vi "Initialize.vi"(4 "Allow Handler Configuration [F]":bool, 5 "HTTP Client In":refnum<class "HttpClient_NET.lvclass">, 7 "AllowedProtocols":i32[](array[ring]) items=["SystemDefault"=0, "Ssl3"=48, "Tls"=192, "Tls11"=768, "Tls12"=3072, "Tls13"=12288], 8 "error in (no error)":errorcluster) -> (0 "error out":errorcluster, 3 "HTTP Client Out":refnum<class "HttpClient_NET.lvclass">)   [LabVIEW 2018, in "HttpClient_NET.lvlib" / "HttpClient_NET.lvclass"]
uses:
  HttpClient_NET.lvclass
  System.Net.Http
  HttpClient_NET.lvclass/HttpClient_NET.ctl
  Accessors/Write NET_HttpClientHandler.vi
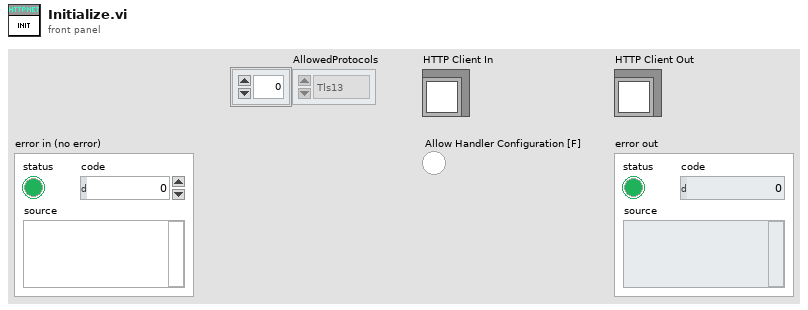
[diagram p1: front panel]
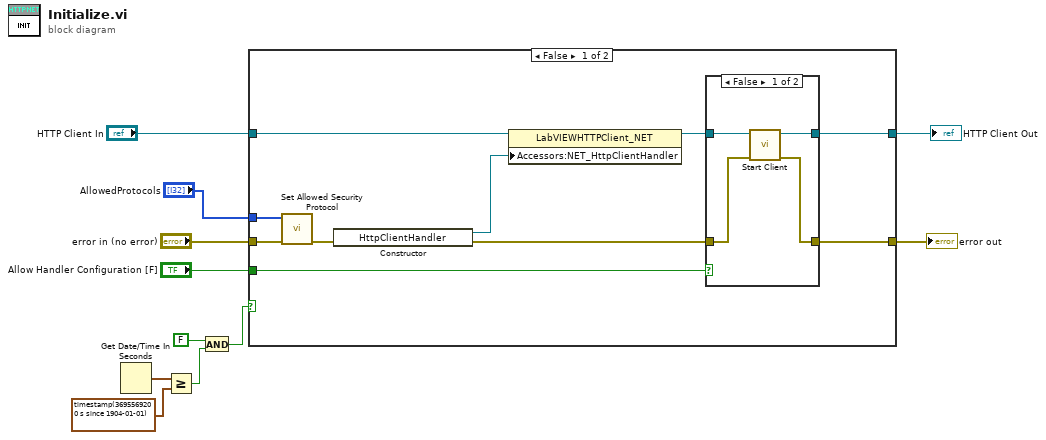
[diagram p0: block diagram]
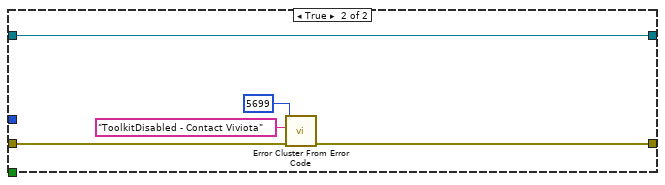
[diagram p3: hidden frame]
diagram:
  n1 = Get Date/Time In Seconds() -> (seconds since 1Jan1904=w5:timestamp)
  n2 = Greater Or Equal?(x=w5, y=timestamp(3695569200 s since 1904-01-01) ("current time")) -> (x >= y?=w3:bool)
  n3 = And(x=FALSE, y=w3) -> (x .and. y?=w2:bool)
  n4 = case shown="False" w2 {
    tunnel: "HTTP Client In" -> [w21 w30]
    tunnel: [w18 w31] -> w10
    tunnel: [w16 w30] -> w9
    tunnel: "Allow Handler Configuration [F]" -> [w15 _]
    tunnel: "error in (no error)" -> [w14 w32]
    tunnel: "AllowedProtocols" -> [w12 _]
    frame False {
      n5 = call "Set Allowed Security Protocol.vi"("error in (no error)"=w14, "AllowedProtocols"=w12) -> ("error out"=w13:errorcluster)  [unwired: 9 in]
      n6 = constructor class="HttpClientHandler"(error in=w13) -> (reference out=w20:refnum<k24>, error out=w19:errorcluster)  [unwired: 2 in, 1 out]
      n7 = property class="LabVIEWHTTPClient_NET"(reference=w21, "Accessors:NET_HttpClientHandler"=w20) -> (reference out=w17:refnum<class "HttpClient_NET.lvclass">)  [unwired: 1 in, 1 out]
      n8 = case shown="False" w15 {
        tunnel: w19 -> [w25 w26]
        tunnel: [w24 w26] -> w18
        tunnel: w17 -> [w23 w27]
        tunnel: [w22 w27] -> w16
        frame False {
          n9 = call "Start Client.vi"("error in (no error)"=w25, "LabVIEWHTTPClient_NET in"=w23) -> ("error out"=w24:errorcluster, "LabVIEWHTTPClient_NET out"=w22:refnum<class "HttpClient_NET.lvclass">)  [unwired: 8 in]
        }
        frame True {
        }
      }
    }
    frame True {
      n10 = call <vilib>:"Error Cluster From Error Code.vi"("error in (no error)"=w32, "error message (\"\")"="ToolkitDisabled - Contact Viviota" ("error message (\"\")"), "error code (0)"=5699) -> ("error out"=w31:errorcluster)  [unwired: 6 in]
    }
  }
  "HTTP Client Out" <- w9
  "error out" <- w10
